vi "AIT 1553 - Create RT Message Name.vi"(0 "RT_Message":T1, 11 "error in (no error)":errorcluster) -> (4 "Message Name":string="CB_R_A_1E_Gun Control", 15 "error out":errorcluster)   [LabVIEW 2013, in "AIT 1553 Custom Device.lvlib"]
uses:
  AIT 1553 Custom Device.lvlib
  Controls/1553_RT_Message.ctl
  Controls/1553 Param.ctl
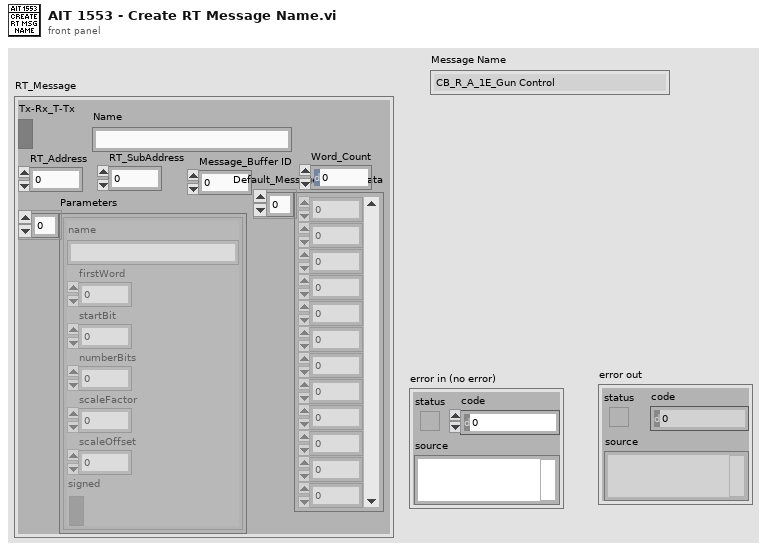
[diagram p1: front panel]
types:
  T1 = typedef "AIT 1553 Custom Device.lvlib/1553_RT_Message.ctl" = cluster{"RT_Address":u8, "RT_SubAddress":u8, "Tx-Rx_T-Tx":bool, "Parameters":T2[], "Message_Buffer ID":u16, "Default_Message_Buffer_Data":u16[], "Word_Count":u8, "Name":string}
  T2 = typedef "AIT 1553 Custom Device.lvlib/1553 Param.ctl" = cluster{"name":string, "firstWord":i32, "startBit":i32, "numberBits":i32, "scaleFactor":dbl, "scaleOffset":dbl, "signed":bool}
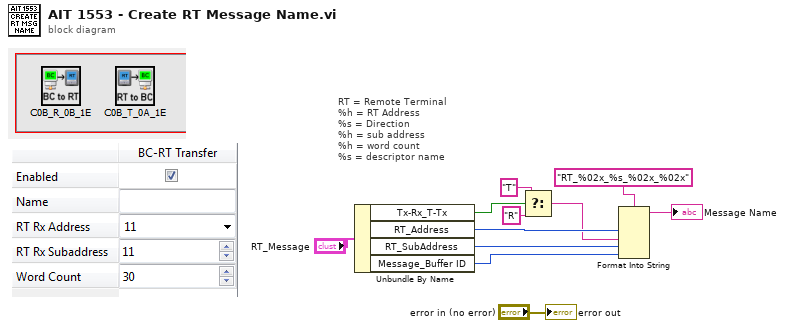
[diagram p0: block diagram]
diagram:
  # "RT = Remote Terminal\n%h = RT Address\n%s = Direction\n%h = sub address\n%h = word count\n%s = descriptor name"
  n1 = Unbundle By Name("RT_Message") -> ("Tx-Rx_T-Tx"=w8:bool, "RT_Address"=w9:u8, "RT_SubAddress"=w3:u8, "Message_Buffer ID"=w4:u16)
  n2 = Select(t="T", s=w8, f="R") -> (s? t:f=w5:string)
  n3 = Format Into String(format string="RT_%02x_%s_%02x_%02x", w9, w5, w3, w4) -> (resulting string=→"Message Name":string)  [unwired: 2 in, 1 out]
  "error out" <- "error in (no error)"
